vi "Add State to Routing Channel.vi"(8 "error in":errorcluster, 10 "state and connections":T1, 11 "routing channel in":T3 format="%.0x") -> (0 "error out":errorcluster, 3 "routing channel out":T3=18446744073709551615 format="%.0x")   [LabVIEW 2020, in "Routing and Faulting Scripting.lvlib"]
doc: "Adds a new state, with a specified configuration, to the routing channel."
uses:
  Routing and Faulting Scripting.lvlib
  <vilib>/NI VeriStand/Custom Device API/Custom Device Item Ref.ctl
  Shared/Routing State.ctl
  Shared/Connection.ctl
  <vilib>/NI VeriStand/Custom Device API/Custom Device API.lvlib
  Dependencies.llb/Routing and Faulting Shared.lvlib
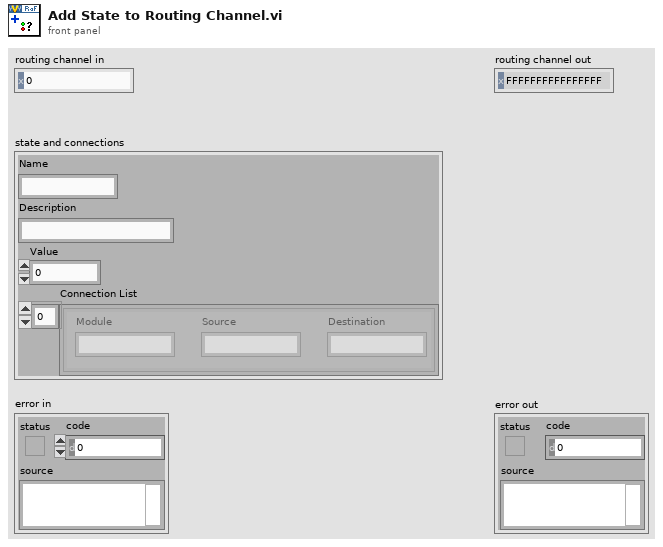
[diagram p1: front panel]
types:
  T1 = typedef "Routing and Faulting Shared.lvlib/Routing State.ctl" = cluster{"Name":string, "Description":string, "Value":i32, "Connection List":T2[]}
  T2 = typedef "Routing and Faulting Shared.lvlib/Connection.ctl" = cluster{"Module":string, "Source":string, "Destination":string}
  T3 = typedef "Custom Device API.lvlib/Custom Device Item Ref.ctl" = u64
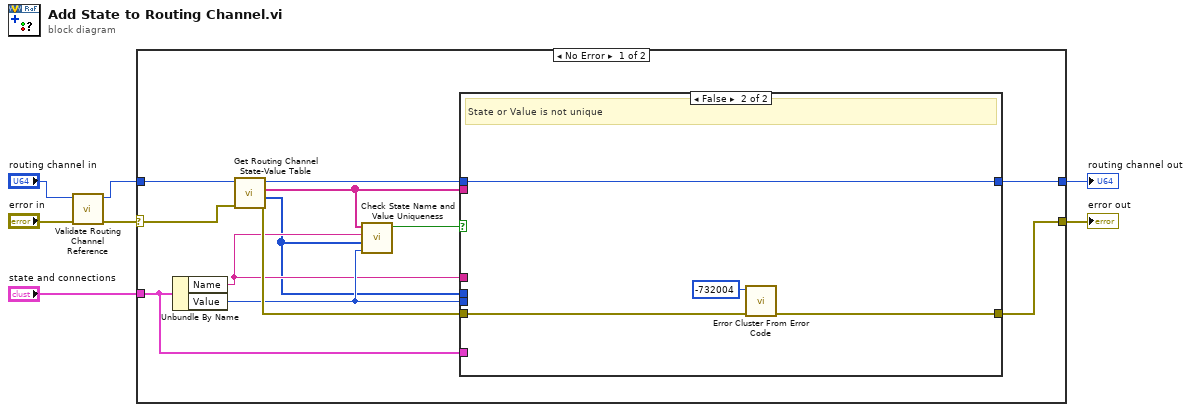
[diagram p0: block diagram]
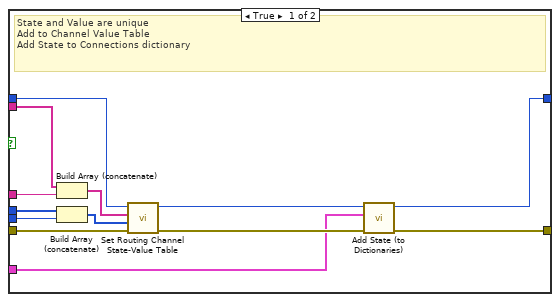
[diagram p2: hidden frame]
diagram:
  n1 = call "Validate Routing Channel Reference.vi"("error in"="error in", "routing channel in"="routing channel in") -> ("error out"=w3:errorcluster, "routing channel out"=w1:T3)  [unwired: 8 in]
  n2 = case shown="No Error" w3 {
    selector: w3 -> [w18 w38]
    tunnel: [w14 w38] -> w5
    tunnel: w1 -> [w19 w37]
    tunnel: [w15 w37] -> w6
    tunnel: "state and connections" -> [w11 _]
    frame No Error {
      n3 = Unbundle By Name(w11) -> ("Name"=w9:string, "Value"=w10:i32)
      n4 = call "Get Routing Channel State-Value Table.vi"("error in"=w18, "routing channel in"=w19) -> ("error out"=w16:errorcluster, "state values"=w8:i32[], "state names"=w13:string[], "routing channel out"=w17:T3)  [unwired: 6 in]
      n5 = call "Check State Name and Value Uniqueness.vi"("value"=w10, "state values"=w8, "name"=w9, "state names"=w13) -> ("is unique"=w12:bool)  [unwired: 7 in]
      n6 = case shown="False" w12 {
        tunnel: w17 -> [w29 w33]
        tunnel: w16 -> [w28 w35]
        tunnel: w8 -> [w31 _]
        tunnel: [w24 w33] -> w15
        tunnel: [w21 w34] -> w14
        tunnel: w10 -> [w32 _]
        tunnel: w13 -> [w30 _]
        tunnel: w9 -> [w23 _]
        tunnel: w11 -> [w20 _]
        frame True {
          # "State and Value are unique\nAdd to Channel Value Table\nAdd State to Connections dictionary"
          n7 = Build Array (concatenate)(w30, w23) -> (w27:string[])
          n8 = Build Array (concatenate)(w31, w32) -> (w26:i32[])
          n9 = call "Set Routing Channel State-Value Table.vi"("error in"=w28, "state values"=w26, "state names"=w27, "routing channel in"=w29) -> ("error out"=w22:errorcluster, "routing channel out"=w25:T3)  [unwired: 6 in]
          n10 = call "Add State (to Dictionaries).vi"("error in"=w22, "state and connections"=w20, "routing channel in"=w25) -> ("error out"=w21:errorcluster, "routing channel out"=w24:T3)  [unwired: 7 in]
        }
        frame False {
          # "State or Value is not unique"
          n11 = call <vilib>:"Error Cluster From Error Code.vi"("error in (no error)"=w35, "error code (0)"=-732004) -> ("error out"=w34:errorcluster)  [unwired: 7 in]
        }
      }
    }
    frame Error {
    }
  }
  "routing channel out" <- w6
  "error out" <- w5
